vi "timer.vi"(8 "error in (no error)":errorcluster, 11 "Delay Time":dbl) -> (0 "error out":errorcluster)   [LabVIEW 2015]
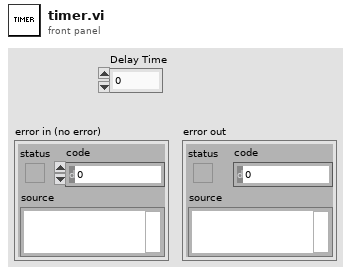
[diagram p1: front panel]
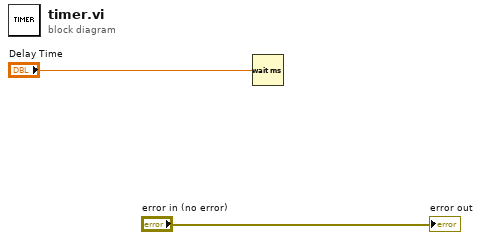
[diagram p0: block diagram]
diagram:
  n1 = Wait (ms)(milliseconds to wait="Delay Time") -> ()  [unwired: 1 out]
  "error out" <- "error in (no error)"
